vi "Comunicación_VFD.vi"(4 "Salidas digitales":bool[](array[boolean]), 6 "Reset":bool, 7 "Frecuencia":dbl, 8 "Sentido":bool, 9 "Run":bool, 10 "Fabricante":u32, 11 "Instancia Modbus":refnum<class "Modbus Master.lvclass">) -> (0 "Error Modbus":errorcluster, 3 "Entradas digitales":bool[](array[boolean]))   [LabVIEW 2013]
uses:
  <vilib>/NI/Modbus Library/API/Master/Modbus Master.lvclass
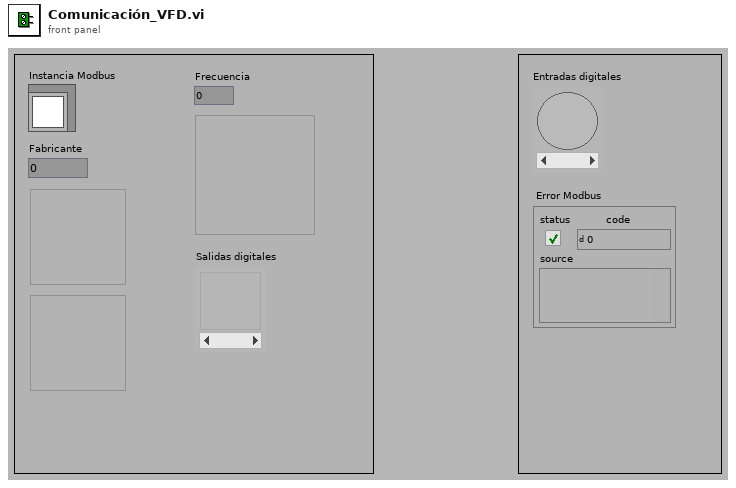
[diagram p1: front panel]
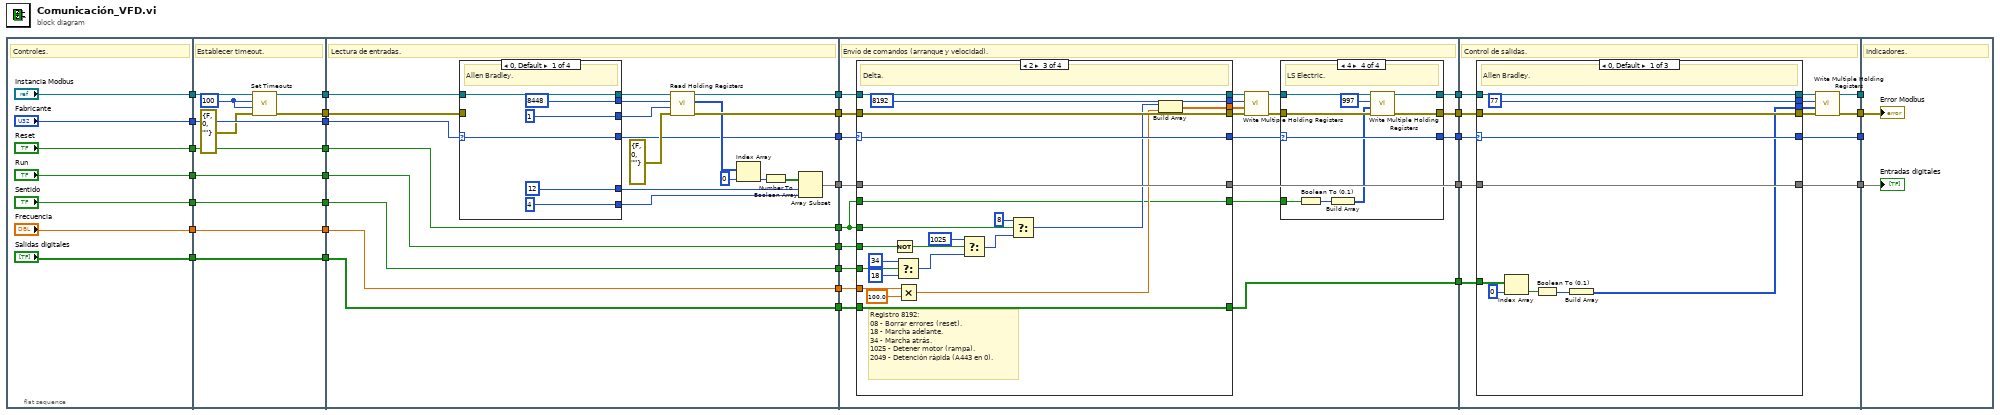
[diagram p0: block diagram]
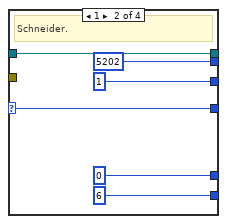
[diagram p2: hidden frame]
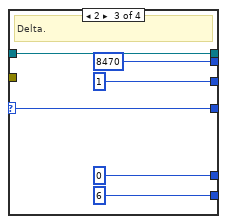
[diagram p3: hidden frame]
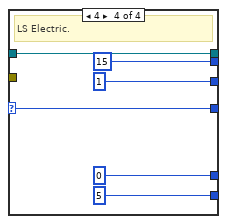
[diagram p4: hidden frame]
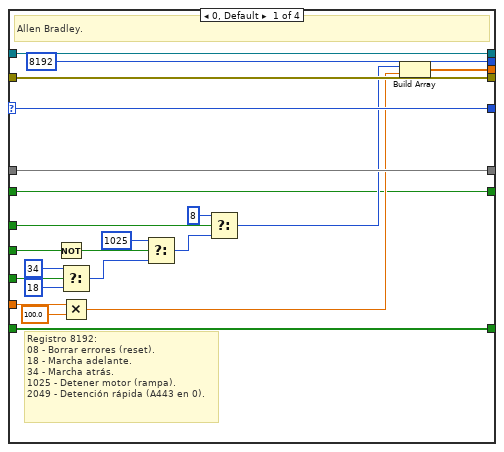
[diagram p8: hidden frame]
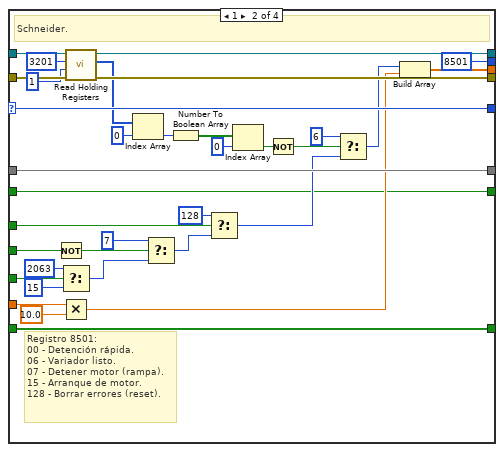
[diagram p9: hidden frame]
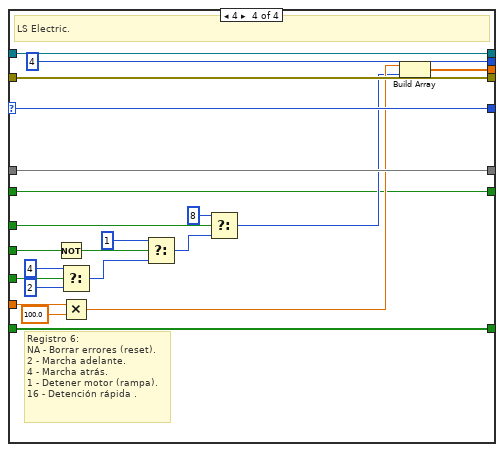
[diagram p10: hidden frame]
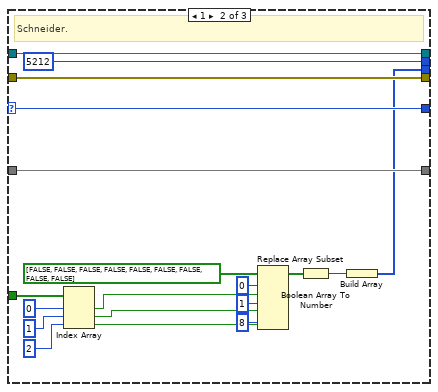
[diagram p11: hidden frame]
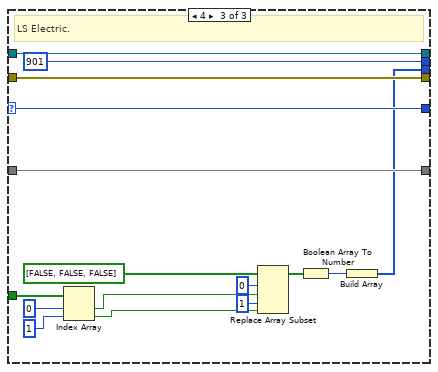
[diagram p12: hidden frame]
diagram:
  n1 = flat-sequence {
    tunnel: ["Instancia Modbus"] -> w15
    tunnel: ["Fabricante"] -> w13
    tunnel: ["Reset"] -> w11
    tunnel: ["Run"] -> w9
    tunnel: ["Sentido"] -> w7
    tunnel: ["Frecuencia"] -> w5
    tunnel: ["Salidas digitales"] -> w3
    tunnel: w15 -> [w45]
    tunnel: [w44] -> w14
    tunnel: w13 -> [w51]
    tunnel: [w51] -> w12
    tunnel: w11 -> [w50]
    tunnel: [w50] -> w10
    tunnel: w9 -> [w49]
    tunnel: [w49] -> w8
    tunnel: w7 -> [w48]
    tunnel: [w48] -> w6
    tunnel: w5 -> [w47]
    tunnel: [w47] -> w4
    tunnel: w3 -> [w46]
    tunnel: [w46] -> w2
    tunnel: [w43] -> w1
    tunnel: w14 -> [w70]
    tunnel: w12 -> [w71]
    tunnel: [w73] -> w33
    tunnel: [w63] -> w32
    tunnel: [w59] -> w31
    tunnel: [w58] -> w30
    tunnel: [w56] -> w29
    tunnel: [w57] -> w28
    tunnel: [w54] -> w27
    tunnel: [w53] -> w19
    tunnel: [w55] -> w17
    tunnel: w10 -> [w57]
    tunnel: w8 -> [w56]
    tunnel: w6 -> [w55]
    tunnel: w4 -> [w54]
    tunnel: w2 -> [w53]
    tunnel: w1 -> [w52]
    tunnel: w33 -> [w116]
    tunnel: [w102] -> w26
    tunnel: w32 -> [w118]
    tunnel: [w104] -> w24
    tunnel: w31 -> [w114]
    tunnel: [w113] -> w23
    tunnel: w30 -> [w119]
    tunnel: w29 -> [w111]
    tunnel: w28 -> [w99]
    tunnel: [w101] -> w21
    tunnel: w27 -> [w109]
    tunnel: w19 -> [w108]
    tunnel: [w107] -> w18
    tunnel: w17 -> [w106]
    tunnel: w26 -> [w245]
    tunnel: [w250] -> w25
    tunnel: w24 -> [w249]
    tunnel: w23 -> [w246]
    tunnel: [w240] -> w22
    tunnel: w21 -> [w247]
    tunnel: [w251] -> w20
    tunnel: w18 -> [w243]
    tunnel: [w239] -> w16
    tunnel: w25 -> [w298]
    tunnel: w22 -> [w297]
    tunnel: w20 -> [_]
    tunnel: w16 -> [_]
    frame #0 {
      # "Controles."
    }
    frame #1 {
      w41 = 100 ("read operation timeout")
      # "Establecer timeout."
      n2 = call <vilib>:"Set Timeouts.vi"("error in"=errorcluster {"status"=FALSE, "code"=0, "source"=""}, "write operation timeout"=w41, "read operation timeout"=w41, "Modbus master in"=w45) -> ("error out"=w43:errorcluster, "Modbus master out"=w44:refnum<class "Modbus Master.lvclass">)  [unwired: 6 in]
    }
    frame #2 {
      # "Lectura de entradas."
      n3 = case shown="0, Default" w71 {
        selector: w71 -> [w76 w82 w88 w94]
        tunnel: w70 -> [w79 w85 w91 w97]
        tunnel: [w79 w85 w91 w97] -> w68
        tunnel: [8448 5202 8470 15] -> w69
        tunnel: [1 1 1 1] -> w67
        tunnel: [w76 w82 w88 w94] -> w58
        tunnel: [12 0 0 0] -> w61
        tunnel: [4 6 6 5] -> w60
        tunnel: w52 -> [_ _ _ _]
        frame 0, Default {
          # "Allen Bradley."
        }
        frame 1 {
          # "Schneider."
        }
        frame 2 {
          # "Delta."
        }
        frame 4 {
          # "LS Electric."
        }
      }
      n4 = call-dynamic "Read Holding Registers.vi"("error in"=errorcluster {"status"=FALSE, "code"=0, "source"=""}, "number of inputs"=w67, "starting address"=w69, "Modbus master in"=w68) -> ("error out"=w73:errorcluster, "register values"=w66:u16[], "Modbus master out"=w63:refnum<class "Modbus Master.lvclass">)  [unwired: 5 in]
      n5 = Index Array(array=w66, index=0) -> (element=w64:u16)
      n6 = Number To Boolean Array(number=w64) -> (Boolean array=w62:bool[])
      n7 = Array Subset(array=w62, index=w61, length=w60) -> (w59:bool[])
    }
    frame #3 {
      # "Envío de comandos (arranque y velocidad)."
      n8 = case shown="2" w119 {
        selector: w119 -> [w157 w193 w214 w236]
        tunnel: w118 -> [w159 w177 w216 w238]
        tunnel: [w159 w176 w216 w238] -> w117
        tunnel: [8192 8501 8192 4] -> w112
        tunnel: [w153 w190 w210 w233] -> w110
        tunnel: [w157 w193 w214 w236] -> w100
        tunnel: w116 -> [w156 w175 w213 w235]
        tunnel: [w156 w174 w213 w235] -> w115
        tunnel: [w155 w192 w212 w234] -> w113
        tunnel: w114 -> [w155 w192 w212 w234]
        tunnel: w111 -> [w151 w188 w208 w231]
        tunnel: w99 -> [w154 w191 w211 w218]
        tunnel: w109 -> [w148 w186 w205 w229]
        tunnel: w108 -> [w145 w184 w202 w227]
        tunnel: [w145 w184 w202 w227] -> w107
        tunnel: w106 -> [w144 w183 w201 w226]
        tunnel: [w138 w160 w195 w217] -> w98
        tunnel: w99 -> [w138 w160 w195 w217]
        frame 0, Default {
          # "Registro 8192:\n08 - Borrar errores (reset).\n18 - Marcha adelante.\n34 - Marcha atrás.\n1025 - Detener motor (rampa).\n2049 - Detención rápida (A443 en 0)."
          # "Allen Bradley."
          n9 = Not(x=w151) -> (.not. x?=w141:bool)
          n10 = Select(t=34, s=w144, f=u16 18) -> (s? t:f=w139:i32)
          n11 = Multiply(x=w148, y=100.0) -> (x*y=w146:dbl)
          n12 = Select(t=u16 1025, s=w141, f=w139) -> (s? t:f=w152:i32)
          n13 = Select(t=8, s=w154, f=w152) -> (s? t:f=w149:i32)
          n14 = Build Array(w149, w146) -> (w153:dbl[])
        }
        frame 1 {
          # "Registro 8501:\n00 - Detención rápida.\n06 - Variador listo.\n07 - Detener motor (rampa).\n15 - Arranque de motor.\n128 - Borrar errores (reset)."
          # "Schneider."
          n15 = Not(x=w188) -> (.not. x?=w180:bool)
          n16 = Select(t=2063, s=w183, f=15) -> (s? t:f=w178:i32)
          n17 = Multiply(x=w186, y=10.0) -> (x*y=w161:dbl)
          n18 = call-dynamic "Read Holding Registers.vi"("error in"=w175, "number of inputs"=u16 1, "starting address"=u16 3201, "Modbus master in"=w177) -> ("error out"=w174:errorcluster, "register values"=w171:u16[], "Modbus master out"=w176:refnum<class "Modbus Master.lvclass">)  [unwired: 5 in]
          n19 = Index Array(array=w171, index=0) -> (element=w169:u16)
          n20 = Select(t=7, s=w180, f=w178) -> (s? t:f=w189:i32)
          n21 = Number To Boolean Array(number=w169) -> (Boolean array=w167:bool[])
          n22 = Select(t=128, s=w191, f=w189) -> (s? t:f=w163:i32)
          n23 = Index Array(array=w167, index=0) -> (element=w166:bool)
          n24 = Not(x=w166) -> (.not. x?=w164:bool)
          n25 = Select(t=6, s=w164, f=w163) -> (s? t:f=w162:i32)
          n26 = Build Array(w162, w161) -> (w190:dbl[])
        }
        frame 2 {
          # "Registro 8192:\n08 - Borrar errores (reset).\n18 - Marcha adelante.\n34 - Marcha atrás.\n1025 - Detener motor (rampa).\n2049 - Detención rápida (A443 en 0)."
          # "Delta."
          n27 = Not(x=w208) -> (.not. x?=w198:bool)
          n28 = Select(t=34, s=w201, f=u16 18) -> (s? t:f=w196:i32)
          n29 = Multiply(x=w205, y=100.0) -> (x*y=w203:dbl)
          n30 = Select(t=u16 1025, s=w198, f=w196) -> (s? t:f=w209:i32)
          n31 = Select(t=8, s=w211, f=w209) -> (s? t:f=w206:i32)
          n32 = Build Array(w206, w203) -> (w210:dbl[])
        }
        frame 4 {
          # "Registro 6:\nNA - Borrar errores (reset).\n2 - Marcha adelante.\n4 - Marcha atrás.\n1 - Detener motor (rampa).\n16 - Detención rápida ."
          # "LS Electric."
          n33 = Not(x=w231) -> (.not. x?=w223:bool)
          n34 = Select(t=4, s=w226, f=2) -> (s? t:f=w221:i32)
          n35 = Multiply(x=w229, y=100.0) -> (x*y=w220:dbl)
          n36 = Select(t=1, s=w223, f=w221) -> (s? t:f=w232:i32)
          n37 = Select(t=8, s=w218, f=w232) -> (s? t:f=w219:i32)
          n38 = Build Array(w220, w219) -> (w233:dbl[])
        }
      }
      n39 = call-dynamic "Write Multiple Holding Registers.vi"("error in"=w115, "registers to write"=w110, "starting address"=w112, "Modbus master in"=w117) -> ("error out"=w103:errorcluster, "Modbus master out"=w105:refnum<class "Modbus Master.lvclass">)  [unwired: 6 in]
      n40 = case shown="4" w100 {
        selector: w100 -> [w121 w124 w127 w137]
        tunnel: w105 -> [w122 w125 w128 w136]
        tunnel: [w122 w125 w128 w135] -> w104
        tunnel: [w121 w124 w127 w137] -> w101
        tunnel: w103 -> [w120 w123 w126 w134]
        tunnel: [w120 w123 w126 w133] -> w102
        tunnel: w98 -> [_ _ _ w131]
        frame 0, Default {
          # "Allen Bradley."
        }
        frame 1 {
          # "Schneider."
        }
        frame 2 {
          # "Delta."
        }
        frame 4 {
          # "LS Electric."
          n41 = Boolean To (0,1)(Boolean=w131) -> (0, 1=w130:i16)
          n42 = Build Array(w130) -> (w129:i16[])
          n43 = call-dynamic "Write Multiple Holding Registers.vi"("error in"=w134, "registers to write"=w129, "starting address"=u16 997, "Modbus master in"=w136) -> ("error out"=w133:errorcluster, "Modbus master out"=w135:refnum<class "Modbus Master.lvclass">)  [unwired: 6 in]
        }
      }
    }
    frame #4 {
      # "Control de salidas."
      n44 = case shown="0, Default" w247 {
        selector: w247 -> [w259 w278 w294]
        tunnel: w249 -> [w261 w280 w296]
        tunnel: [w261 w280 w296] -> w248
        tunnel: [77 5212 901] -> w244
        tunnel: [w259 w278 w294] -> w239
        tunnel: w246 -> [w258 w277 w293]
        tunnel: [w258 w277 w293] -> w240
        tunnel: w245 -> [w255 w274 w290]
        tunnel: w243 -> [w257 w276 w292]
        tunnel: [w255 w274 w290] -> w242
        tunnel: [w252 w273 w289] -> w241
        frame 0, Default {
          # "Allen Bradley."
          n45 = Index Array(array=w257, index=0) -> (element=w254:bool)
          n46 = Boolean To (0,1)(Boolean=w254) -> (0, 1=w253:i16)
          n47 = Build Array(w253) -> (w252:i16[])
        }
        frame 1 {
          # "Schneider."
          n48 = Index Array(array=w276, index #1=0 ("index"), index #2=1 ("index"), index #3=2 ("index")) -> (element #1=w268:bool, element #2=w267:bool, element #3=w262:bool)
          n49 = Replace Array Subset(array=bool[] [FALSE, FALSE, FALSE, FALSE, FALSE, FALSE, FALSE, FALSE, FALSE], new element #1=w268, index #1=0 ("index"), new element #2=w267, index #2=1 ("index"), new element #3=w262, index #3=8 ("index")) -> (w270:bool[])
          n50 = Boolean Array To Number(Boolean array=w270) -> (number=w269:u32)
          n51 = Build Array(w269) -> (w273:u32[])
        }
        frame 4 {
          # "LS Electric."
          n52 = Index Array(array=w292, index #1=0 ("index"), index #2=1 ("index")) -> (element #1=w285:bool, element #2=w284:bool)
          n53 = Replace Array Subset(array=bool[] [FALSE, FALSE, FALSE], new element #1=w285, index #1=0 ("index"), new element #2=w284, index #2=1 ("index")) -> (w287:bool[])
          n54 = Boolean Array To Number(Boolean array=w287) -> (number=w286:u32)
          n55 = Build Array(w286) -> (w289:u32[])
        }
      }
      n56 = call-dynamic "Write Multiple Holding Registers.vi"("error in"=w242, "registers to write"=w241, "starting address"=w244, "Modbus master in"=w248) -> ("error out"=w250:errorcluster, "Modbus master out"=w251:refnum<class "Modbus Master.lvclass">)  [unwired: 6 in]
    }
    frame #5 {
      # "Indicadores."
      "Error Modbus" <- w298
      "Entradas digitales" <- w297
    }
  }
